vi "get_relative_frame.vi"(8 "error in (no error)":errorcluster, 9 "relative depth":dbl[unit], 10 "relative time":dbl[unit], 11 "ImageCollection in":refnum<class "ImageCollection.lvclass">) -> (0 "error out":errorcluster, 1 "difference":dbl[unit], 2 "frame":refnum<class "Image.lvclass">, 3 "ImageCollection out":refnum<class "ImageCollection.lvclass">)   [LabVIEW 2010, in "ImageCollection.lvclass"]
uses:
  ImageCollection.lvclass
  Image/Image/Image.lvclass
  add_mode_enum.ctl
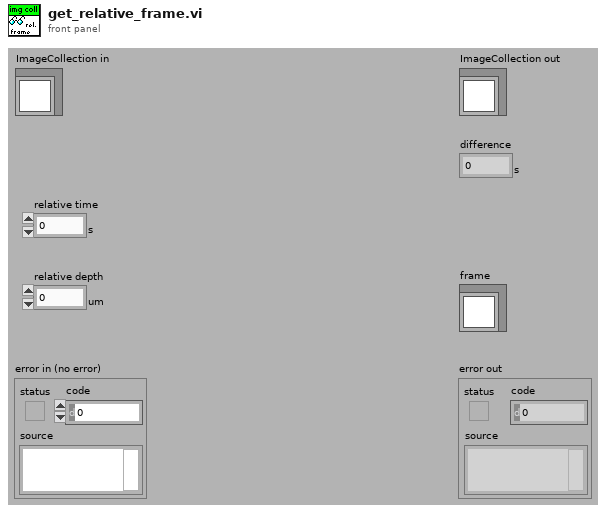
[diagram p1: front panel]
types:
  T1 = typedef "ImageCollection.lvclass/add_mode_enum.ctl" = enum16{"instance", "copy"}
  T2 = typedef "type_enum.ctl" = enum16{"undefined", "movie", "z-stack"}
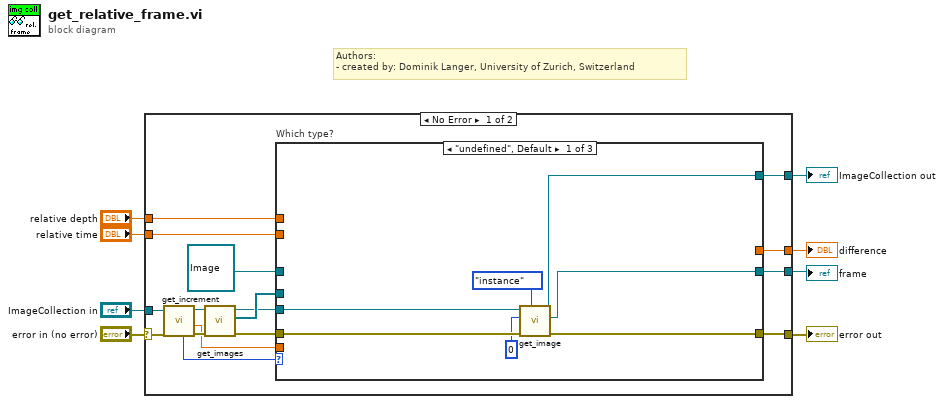
[diagram p0: block diagram]
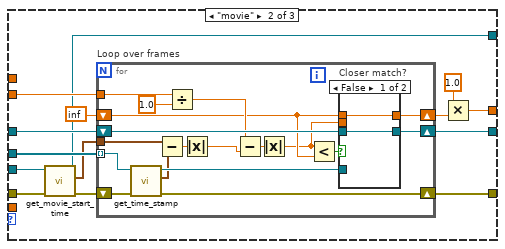
[diagram p2: hidden frame]
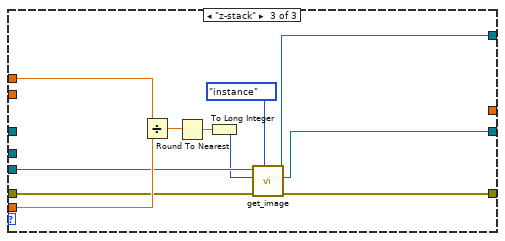
[diagram p4: hidden frame]
diagram:
  # "Authors: \n- created by: Dominik Langer, University of Zurich, Switzerland"
  n1 = case shown="No Error" "error in (no error)" {
    selector: "error in (no error)" -> [w12 w80]
    tunnel: [w22 w80] -> w7
    tunnel: [w13 w79] -> w5
    tunnel: "ImageCollection in" -> [w11 w79]
    tunnel: "relative time" -> [w20 _]
    tunnel: [w18 _] -> w3
    tunnel: [w19 _] -> w2
    tunnel: "relative depth" -> [w10 _]
    frame No Error {
      n2 = call "get_increment.vi"("error in (no error)"=w12, "ImageCollection in"=w11) -> ("error out"=w17:errorcluster, "z increment"=w9:dbl[unit], "ImageCollection out"=w16:refnum<class "ImageCollection.lvclass">, "type"=w15:T2)  [unwired: 5 in, 1 out]
      n3 = call-dynamic "get_images.vi"("error in (no error)"=w17, "ImageCollection.lvclass in"=w16) -> ("error out"=w24:errorcluster, "images"=w23:refnum<class "Image.lvclass">[], "ImageCollection.lvclass out"=w14:refnum<class "ImageCollection.lvclass">)  [unwired: 7 out]
      n4 = case "Which type?" shown="\"undefined\", Default" w15 {
        tunnel: w24 -> [w31 w36 w74]
        tunnel: w23 -> [_ w45 _]
        tunnel: [w30 w44 w71] -> w22
        tunnel: refnum<class "Image.lvclass"> refnum ("Image.lvclass") -> [_ w43 _]
        tunnel: w20 -> [_ w42 _]
        tunnel: [w25 w41 w68] -> w19
        tunnel: [_ w38 _] -> w18
        tunnel: w14 -> [w29 w34 w73]
        tunnel: [w28 w33 w72] -> w13
        tunnel: w10 -> [_ _ w78]
        tunnel: w9 -> [_ _ w77]
        frame "undefined", Default {
          n5 = call-dynamic "get_image.vi"("get image as..."=add_mode_enum."instance", "error in (no error)"=w31, "index"=0, "ImageCollection in"=w29) -> ("error out"=w30:errorcluster, "Image.lvclass"=w25:refnum<class "Image.lvclass">, "ImageCollection out"=w28:refnum<class "ImageCollection.lvclass">)  [unwired: 5 in]
        }
        frame "movie" {
          n6 = call-dynamic "get_movie_start_time.vi"("error in (no error)"=w36, "ImageCollection.lvclass in"=w34) -> ("error out"=w35:errorcluster, "movie start"=w32:timestamp, "ImageCollection.lvclass out"=w33:refnum<class "ImageCollection.lvclass">)  [unwired: 7 out]
          n7 = for "Loop over frames" {
            tunnel: w45 -> [w62] mode=indexing
            shift-right: [w60] -> w44
            shift-left: w35 -> [w63]
            tunnel: w32 -> [w61]
            shift-right: [w56] -> w39
            shift-left: inf -> [w48]
            shift-right: [w58] -> w41
            shift-left: w43 -> [w59]
            tunnel: w42 -> [w53]
            n8 = call-dynamic "get_time_stamp.vi"("error in (no error)"=w63, "Image.lvclass in"=w62) -> ("error out"=w60:errorcluster, "timestamp"=w55:timestamp, "Image.lvclass out"=w57:refnum<class "Image.lvclass">)  [unwired: 7 out]
            n9 = Subtract(x=w61, y=w55) -> (x-y=w54:dbl)
            n10 = Divide(x=w53, y=dbl[unit] 1.0) -> (x/y=w52:dbl)
            n11 = Absolute Value(x=w54) -> (abs(x)=w49:dbl)
            n12 = Subtract(x=w52, y=w49) -> (x-y=w47:dbl)
            n13 = Absolute Value(x=w47) -> (abs(x)=w46:dbl)
            n14 = Less?(x=w46, y=w48) -> (x < y?=w50:bool)
            n15 = case "Closer match?" shown="False" w50 {
              tunnel: w59 -> [w65 _]
              tunnel: [w65 w67] -> w58
              tunnel: w57 -> [_ w67]
              tunnel: w48 -> [w64 _]
              tunnel: [w64 w66] -> w56
              tunnel: w46 -> [_ w66]
              frame False {
              }
              frame True {
              }
            }
          }
          n16 = Multiply(x=dbl[unit] 1.0, y=w39) -> (x*y=w38:dbl[unit])
        }
        frame "z-stack" {
          n17 = Divide(x=w78, y=w77) -> (x/y=w76:dbl)
          n18 = Round To Nearest(number=w76) -> (nearest integer value=w75:dbl)
          n19 = To Long Integer(number=w75) -> (32bit integer=w69:i32)
          n20 = call-dynamic "get_image.vi"("get image as..."=add_mode_enum."instance", "error in (no error)"=w74, "index"=w69, "ImageCollection in"=w73) -> ("error out"=w71:errorcluster, "Image.lvclass"=w68:refnum<class "Image.lvclass">, "ImageCollection out"=w72:refnum<class "ImageCollection.lvclass">)  [unwired: 5 in]
        }
      }
    }
    frame Error {
    }
  }
  "error out" <- w7
  "ImageCollection out" <- w5
  "difference" <- w3
  "frame" <- w2
